vi "poll data.vi"(8 "error in (no error)":errorcluster caption="错误输入（无错误）", 11 "BD Protocol 4.0 输入":refnum<class "BD Protocol 4.0.lvclass">) -> (0 "error out":errorcluster caption="错误输出", 3 "BD Protocol 4.0 输出":refnum<class "BD Protocol 4.0.lvclass">)   [LabVIEW 2016, in "BD Protocol 4.0.lvlib" / "BD Protocol 4.0.lvclass"]
uses:
  BD Protocol 4.0.lvclass
  BD Protocol 4.0.lvclass/BD Protocol 4.0.ctl
  <vilib>/regexp/Match Regular Expression.xnode
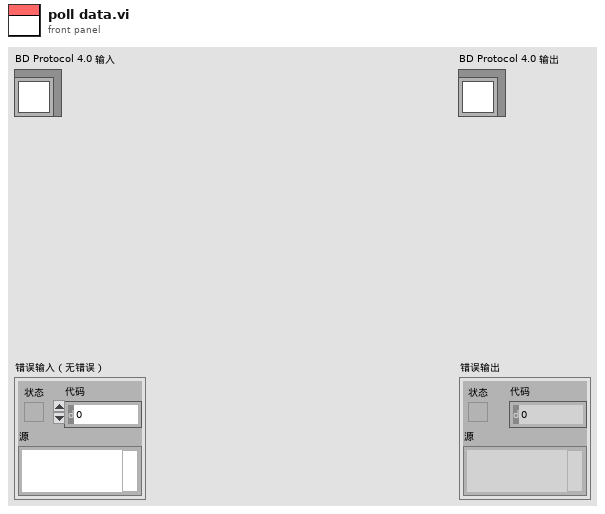
[diagram p1: front panel]
types:
  T1 = cluster{"指令":string, "长度":u16, "用户地址":string, "信息内容":cluster{"信息类别":u8, "发信方地址":string, "发信时间时":u8, "发信时间分":u8, "长度":u16, "电文内容":string, "CRC标志":u8}, "校验和":u8}
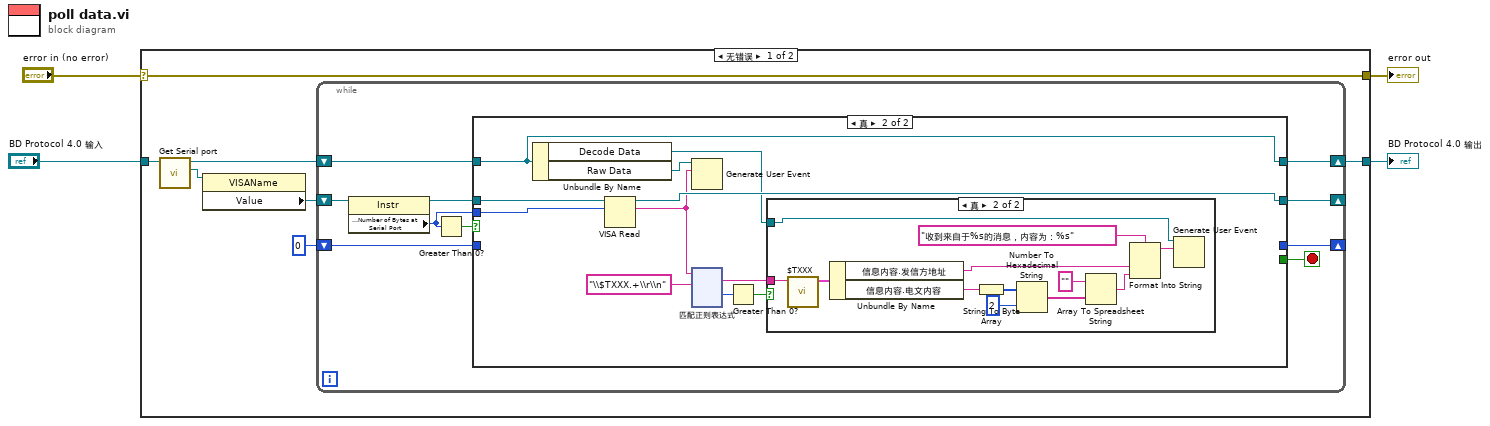
[diagram p0: block diagram]
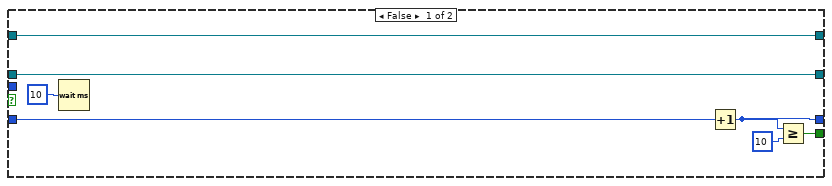
[diagram p2: hidden frame]
diagram:
  n1 = case shown="无错误" "error in (no error)" {
    selector: "error in (no error)" -> [w11 w167]
    tunnel: [w11 w167] -> w3
    tunnel: [w5 w166] -> w1
    tunnel: "BD Protocol 4.0 输入" -> [w10 w166]
    frame No Error {
      n2 = call "Get Serial port.vi"("BD Protocol 4.0 in"=w10) -> ("Serial port"=w9:refnum<vi>, "BD Protocol 4.0 out"=w7:refnum<class "BD Protocol 4.0.lvclass">)  [unwired: 9 in]
      n3 = property class="VISAName"(reference=w9) -> ("Value"=w8:refnum<visa-resource-name>)  [unwired: 1 in, 2 out]
      n4 = while {
        shift-right: [w17] -> _
        shift-left: w8 -> [w21]
        shift-right: [w14] -> _
        shift-left: 0 -> [w15]
        shift-right: [w12] -> w5
        shift-left: w7 -> [w16]
        stop <- w13 stop-if-true
        n5 = property class="Instr"(reference=w21) -> (reference out=w19:refnum<visa-resource-name>, "Serial Settings:Number of Bytes at Serial Port"=w18:u32)  [unwired: 1 in, 1 out]
        n6 = Greater Than 0?(x=w18) -> (x > 0?=w20:bool)
        n7 = case shown="真" w20 {
          tunnel: w19 -> [w28 w39]
          tunnel: w18 -> [_ w38]
          tunnel: [w28 w37] -> w17
          tunnel: w16 -> [w22 w35]
          tunnel: w15 -> [w26 _]
          tunnel: [w25 _] -> w14
          tunnel: [w23 _] -> w13
          tunnel: [w22 w35] -> w12
          frame False {
            n8 = Wait (ms)(milliseconds to wait=u32 10 ("等待时间（毫秒）")) -> ()  [unwired: 1 out]
            n9 = Increment(x=w26) -> (x+1=w25:i32)
            n10 = Greater Or Equal?(x=w25, y=10) -> (x >= y?=w23:bool)
          }
          frame True {
            n11 = Unbundle By Name(w35) -> ("Decode Data"=w32:refnum<user-event>, "Raw Data"=w36:refnum<user-event>)
            n12 = VISA Read(VISA resource name=w39, byte count=w38) -> (VISA resource name out=w37:refnum<visa-resource-name>, read buffer=w30:string)  [unwired: 1 in, 2 out]
            n13 = Generate User Event(user event=w36, event data cluster=w30) -> ()  [unwired: 2 in, 2 out]
            n14 = xnode "匹配正则表达式"("输入字符串"=w30, "正则表达式"="\\$TXXX.+\\r\\n") -> ("所有匹配"=w31:string, "匹配后偏移量"=w29:i32)  [unwired: 4 in, 3 out]
            n15 = Greater Than 0?(x=w29) -> (x > 0?=w33:bool)
            n16 = case shown="真" w33 {
              tunnel: w32 -> [_ w165]
              tunnel: w31 -> [_ w164]
              frame False {
              }
              frame True {
                n17 = call "$TXXX.vi"("反馈信息"=w164) -> ("接收信息"=w163:T1)  [unwired: 10 in]
                n18 = Unbundle By Name(w163) -> ("信息内容.发信方地址"=w162:string, "信息内容.电文内容"=w161:string)
                n19 = String To Byte Array(string=w161) -> (unsigned byte array=w160:u8[])
                n20 = Number To Hexadecimal String(1:i16 2 ("宽度(-)"), 2:w160) -> (0:w159:string[])
                n21 = Array To Spreadsheet String(array=w159, 3:"" ("格式字符串")) -> (spreadsheet string=w157:string)  [unwired: 1 in]
                n22 = Format Into String(format string="收到来自于%s的消息，内容为：%s" ("格式字符串"), w162, w157) -> (resulting string=w156:string)  [unwired: 2 in, 1 out]
                n23 = Generate User Event(user event=w165, event data cluster=w156) -> ()  [unwired: 2 in, 2 out]
              }
            }
          }
        }
      }
    }
    frame Error {
    }
  }
  "error out" <- w3
  "BD Protocol 4.0 输出" <- w1
